vi "Init PWM.vi"(5 "Phase-Correct (F)":bool, 7 "GPIO":i32, 8 "error in (no error)":errorcluster, 10 "Enable (F)":bool, 11 "VISA resource name in":refnum<visa-resource-name>) -> (0 "error out":errorcluster, 3 "VISA resource name":refnum<visa-resource-name>)   [LabVIEW 2023, in "CTI-Visa.lvlib"]
uses:
  CTI-Visa.lvlib
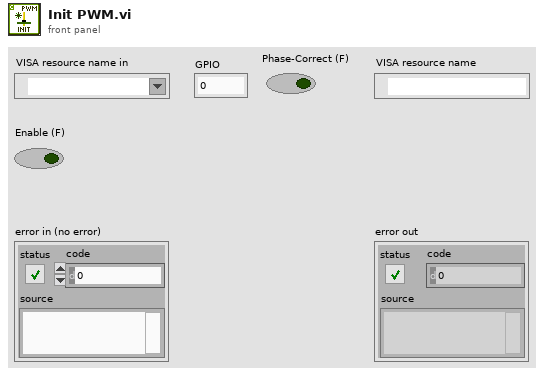
[diagram p1: front panel]
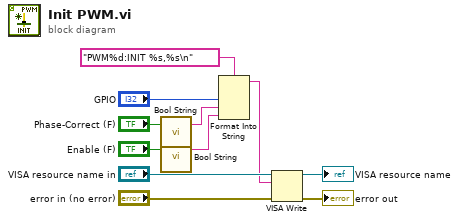
[diagram p0: block diagram]
diagram:
  n1 = call "Bool String.vi"("Bool"="Phase-Correct (F)") -> ("String"=w8:string)  [unwired: 6 in]
  n2 = call "Bool String.vi"("Bool"="Enable (F)") -> ("String"=w7:string)  [unwired: 6 in]
  n3 = Format Into String(format string="PWM%d:INIT %s,%s\n", "GPIO", w8, w7) -> (resulting string=w1:string)  [unwired: 2 in, 1 out]
  n4 = VISA Write(VISA resource name="VISA resource name in", write buffer=w1, error in (no error)="error in (no error)") -> (VISA resource name out=→"VISA resource name":refnum<visa-resource-name>, error out=→"error out":errorcluster)  [unwired: 1 out]
